vi "test Create Connect Message Single Routing Channel State Unchanged.vi"(8 "error in (no error)":errorcluster, 11 "TestCase in":refnum<class "Routing and Faulting Unit Tests.lvclass">) -> (0 "error out":errorcluster, 3 "TestCase out":refnum<class "Routing and Faulting Unit Tests.lvclass">)   [LabVIEW 2017, in "Routing and Faulting Unit Tests.lvclass"]
uses:
  Routing and Faulting Unit Tests.lvclass
  Engine/Engine Data.ctl
  Shared/Compiled.Settings.ctl
  Shared/Communication Configuration.ctl
  Shared/Routing and Faulting Configuration.ctl
  Shared/Routing Channel Configuration.ctl
  Shared/Value-Connections Map.ctl
  Shared/Connection.ctl
  Shared/Alias Mapping.ctl
  Shared/FIFO Indices.ctl
  Includes/CDMessaging.lvlibp/Producer/Abstract Producer/Abstract Producer.lvclass
  Engine/Device Inputs.ctl
  Engine/Device Outputs.ctl
  Engine/Producer Message.ctl
  Includes/CDMessaging.lvlibp/Message/Abstract Message/Abstract Message.lvclass
  <vilib>/addons/_JKI Toolkits/VI Tester/TestCase.llb/TestCase.lvclass
  Engine/Routing and Faulting Engine.lvlib
  Shared/Routing and Faulting Shared.lvlib
  C:/Program Files (x86)/National Instruments/LabVIEW 2017/vi.lib/addons/_JKI Toolkits/VI Tester/TestCase.llb/TestCase.lvclass
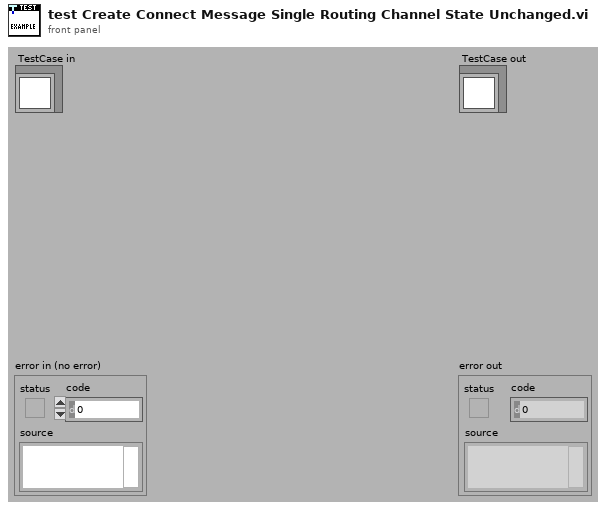
[diagram p1: front panel]
types:
  T1 = typedef "Routing and Faulting Engine.lvlib/Producer Message.ctl" = cluster{"Consumer":string, "Message":refnum<class "Abstract Message.lvclass">}
  T2 = typedef "Routing and Faulting Shared.lvlib/Communication Configuration.ctl" = cluster{"Consumer Queue Names":string[], "Resource Names":string[]}
  T3 = typedef "Routing and Faulting Shared.lvlib/Routing Channel Configuration.ctl" = cluster{"Channel Name":string, "Initial Value":dbl, "FIFO Index":i32, "Value-Connections Map":T4}
  T4 = typedef "Routing and Faulting Shared.lvlib/Value-Connections Map.ctl" = cluster{"State Value Array":i32[], "Connection List Array":cluster{"Connection List":T5[]}[]}
  T5 = typedef "Routing and Faulting Shared.lvlib/Connection.ctl" = cluster{"Resource":string, "Source":string, "Destination":string}
  T6 = typedef "Routing and Faulting Shared.lvlib/Routing and Faulting Configuration.ctl" = cluster{"Routing Channel Configurations":T3[], "Alias Mappings":T7[]}
  T7 = typedef "Routing and Faulting Shared.lvlib/Alias Mapping.ctl" = cluster{"Endpoint":string, "Alias":string}
  T8 = typedef "Routing and Faulting Engine.lvlib/Engine Data.ctl" = cluster{"Compiled.Settings":T9, "Producer":refnum<class "Abstract Producer.lvclass">, "Device Inputs":T11, "Device Outputs":T12, "States Changed":bool[]}
  T9 = typedef "Routing and Faulting Shared.lvlib/Compiled.Settings.ctl" = cluster{"Custom Device Name":string, "Communication Configuration":T2, "Routing and Faulting Configuration":T6, "Status Channels FIFO Indices":T10}
  T10 = typedef "Routing and Faulting Shared.lvlib/FIFO Indices.ctl" = cluster{"Status Channel":i32, "Heartbeat Channel":i32}
  T11 = typedef "Routing and Faulting Engine.lvlib/Device Inputs.ctl" = cluster{"Current Inputs":dbl[], "Previous Inputs":dbl[], "Device Inputs FIFO":refnum<k33>}
  T12 = typedef "Routing and Faulting Engine.lvlib/Device Outputs.ctl" = cluster{"Outputs":dbl[], "Device Outputs FIFO":refnum<k33>}
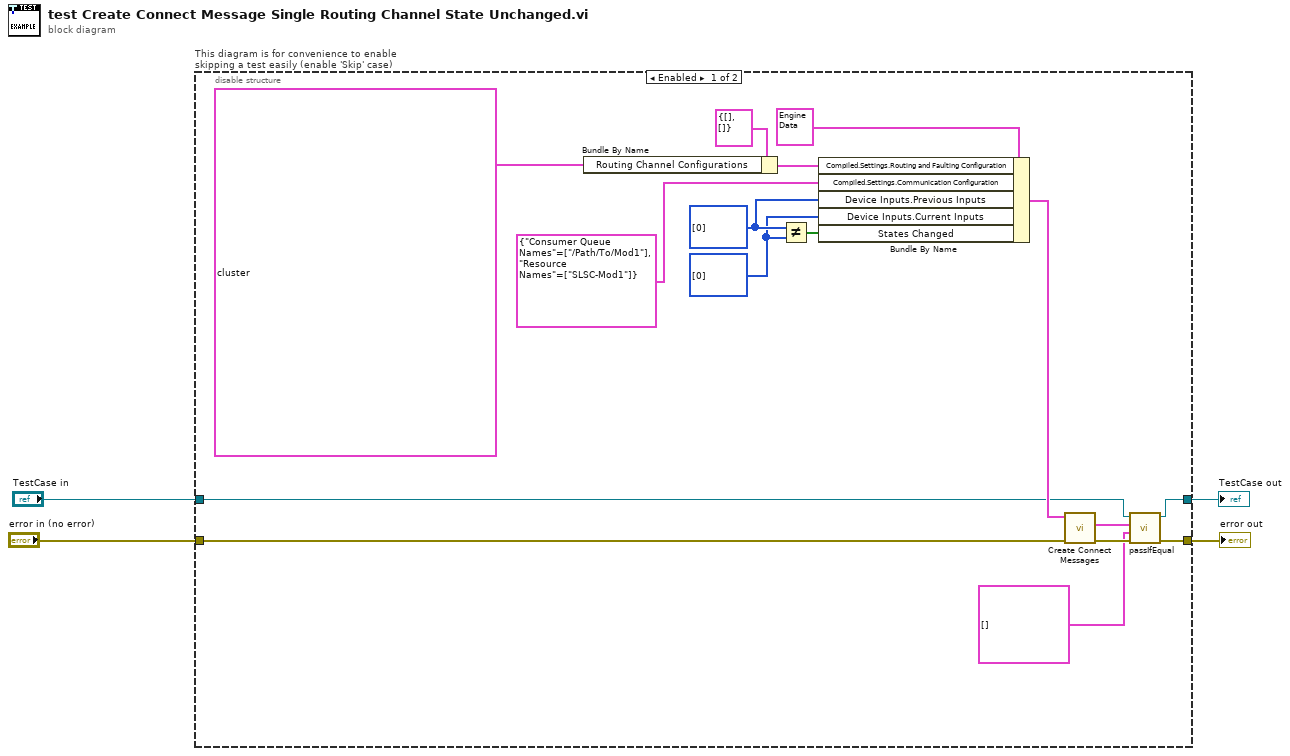
[diagram p0: block diagram]
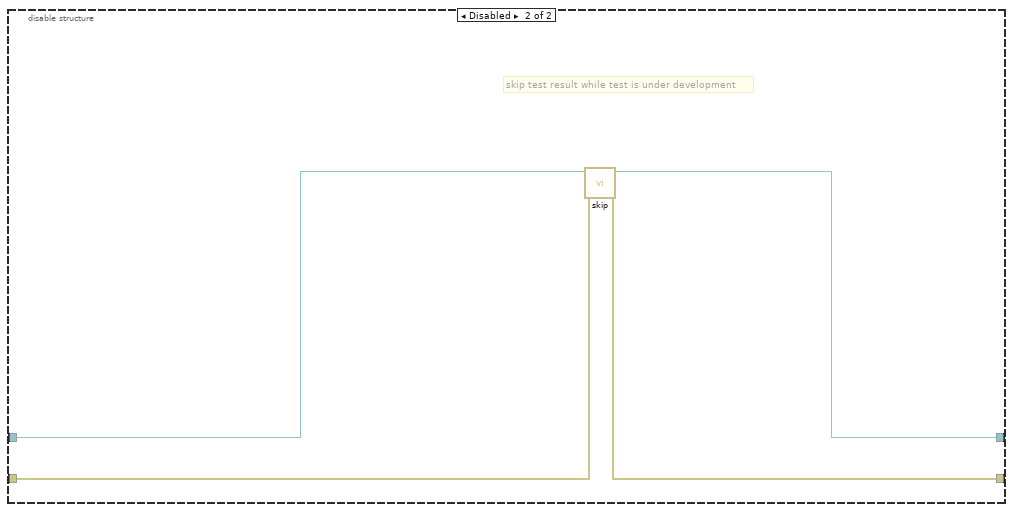
[diagram p2: hidden frame]
diagram:
  n1 = disable-structure "This diagram is for convenience to enable skipping a test easily (enable 'Skip' case)" shown="Enabled" {
    disable-tunnel: "TestCase in" -> [w8 w24]
    disable-tunnel: [w9 w22] -> w1
    disable-tunnel: [w10 w23] -> w3
    disable-tunnel: "error in (no error)" -> [w6 w21]
    frame Enabled {
      w15 = i32[] [0] ("State Value Array")
      w16 = i32[] [0] ("State Value Array")
      n2 = Bundle By Name(cluster=T6 {"Routing Channel Configurations"=[], "Alias Mappings"=[]} ("Compiled.Settings.Routing and Faulting Configuration"), "Routing Channel Configurations"=T3[] [{"Channel Name"="Window Up", "Initial Value"=0.0, "FIFO Index"=0, "Value-Connections Map"={"State Value Array"=[0, 10], "Connection List Array"=[{"Connection List"=[]}, {"Connection List"=[{"Resource"="SLSC-Mod1", "Source"="Ch0", "Destination"="Ch1"}]}]}}]) -> (w18:T6)
      n3 = Not Equal?(x=w16, y=w15) -> (x != y?=w14:bool[])
      n4 = Bundle By Name(cluster=T8 {"Compiled.Settings"={"Custom Device Name"="", "Communication Configuration"={"Consumer Queue Names"=[], "Resource Names"=[]}, "Routing and Faulting Configuration"={"Routing Channel Configurations"=[], "Alias Mappings"=[]}, "Status Channels FIFO Indices"={"Status Channel"=0, "Heartbeat Channel"=0}}, "Producer"=refnum, "Device Inputs"={"Current Inputs"=[], "Previous Inputs"=[], "Device Inputs FIFO"=refnum}, "Device Outputs"={"Outputs"=[], "Device Outputs FIFO"=refnum}, "States Changed"=[]} ("Engine Data in"), "Compiled.Settings.Routing and Faulting Configuration"=w18, "Compiled.Settings.Communication Configuration"=T2 {"Consumer Queue Names"=["/Path/To/Mod1"], "Resource Names"=["SLSC-Mod1"]}, "Device Inputs.Previous Inputs"=w16, "Device Inputs.Current Inputs"=w15, "States Changed"=w14) -> (w12:T8)
      n5 = call "Create Connect Messages.vi"("error in (no error)"=w6, "Engine Data in"=w12) -> ("error out"=w11:errorcluster, "Connect Messages"=w7:T1[])  [unwired: 7 in, 1 out]
      n6 = call-dynamic "passIfEqual.vi"("error in (no error)"=w11, "y"=T1[] [] ("appended array"), "x"=w7, "TestCase in"=w8) -> ("error out"=w10:errorcluster, "TestCase out"=w9:refnum<class "Routing and Faulting Unit Tests.lvclass">)  [unwired: 6 in]
    }
    frame Disabled {
      # "skip test result while test is under development"
      n7 = call <vilib>:"skip.vi"("error in (no error)"=w21, "TestCase in"=w24) -> ("error out"=w23:errorcluster, "TestCase out"=w22:refnum<class "Routing and Faulting Unit Tests.lvclass">)  [unwired: 8 in]
    }
  }
  "error out" <- w3
  "TestCase out" <- w1
